vi "FindWindowA.vi"(8 "error in":errorcluster, 9 "lpszWindowName":string, 10 "lpszClassName":i32(ring) items=["NULL"]) -> (0 "error out":errorcluster, 1 "lpszWindowName Out":string, 2 "lpszClassName Out":i32, 3 "hWnd":u32)   [LabVIEW 2014]
uses:
  user32.dll
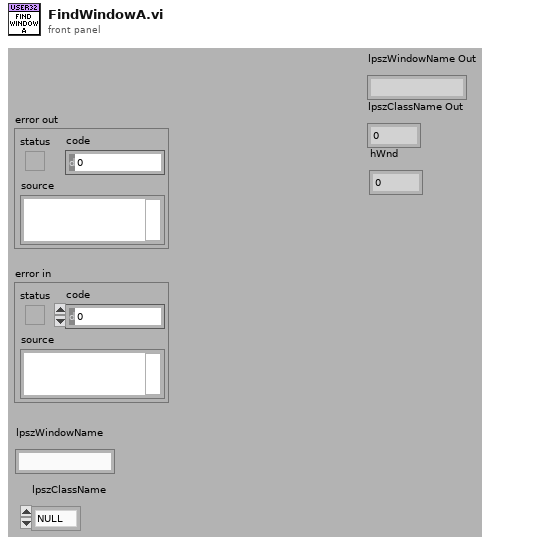
[diagram p1: front panel]
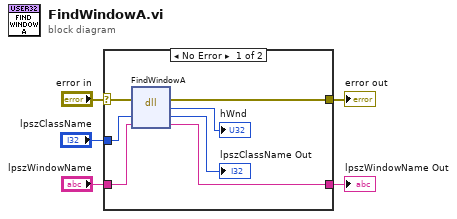
[diagram p0: block diagram]
diagram:
  n1 = case shown="No Error" "error in" {
    selector: "error in" -> [w6 w14]
    tunnel: "lpszWindowName" -> [w12 w13]
    tunnel: [w11 w14] -> w4
    tunnel: "lpszClassName" -> [w10 _]
    tunnel: [w9 w13] -> w2
    frame No Error {
      n2 = dll-call lib="user32.dll" fn="FindWindowA" label="FindWindow"(error in=w6, "lpszClassName"=w10, "lpszWindowName"=w12) -> (error out=w11:errorcluster, "hWnd"=→"hWnd":u32, "lpszClassName"=→"lpszClassName Out":i32, "lpszWindowName"=w9:string)  [unwired: 2 in, 1 out]
    }
    frame Error {
    }
  }
  "error out" <- w4
  "lpszWindowName Out" <- w2
